vi "addExtension.vi"(9 "Extension":string, 11 "In path":path) -> (1 "Out path":string, 3 "Out path":path)   [LabVIEW 2023]
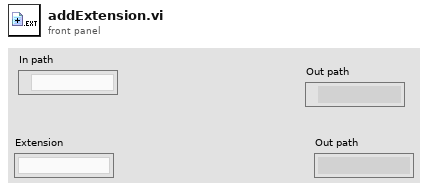
[diagram p1: front panel]
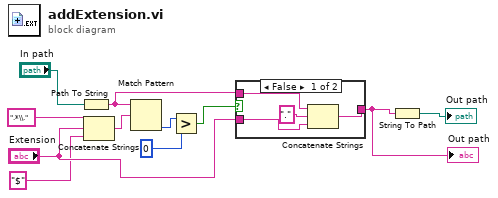
[diagram p0: block diagram]
diagram:
  n1 = Path To String(path="In path") -> (string=w8:string)
  n2 = Concatenate Strings(".*\\." ("string"), "Extension", "$" ("string")) -> (w4:string)
  n3 = Match Pattern(string=w8, regular expression=w4) -> (offset past match=w5:i32)  [unwired: 1 in, 3 out]
  n4 = Greater?(x=w5, y=0) -> (0:w6:bool)
  n5 = case shown="False" w6 {
    tunnel: [w15 w16] -> w9
    tunnel: w8 -> [w13 w16]
    tunnel: "Extension" -> [w12 _]
    frame False {
      n6 = Concatenate Strings(w13, "." ("string"), w12) -> (w15:string)
    }
    frame True {
    }
  }
  "Out path" <- w9
  n7 = String To Path(string=w9) -> (path=→"Out path":path)
